vi "Values.vi"(11 "User in":refnum<class "User.lvclass">) -> (2 "Values":T1)   [LabVIEW 2022 SP3, in "Test.lvlib" / "User.lvclass"]
uses:
  User.lvclass
  Values.ctl
  User.lvclass/User.ctl
  <vilib>/IlluminatedG/IG Conditum/Conditum/Columns/String/String.lvclass/String.ctl
  <vilib>/IlluminatedG/IG Conditum/Conditum/Columns/Timestamp/Timestamp.lvclass/Timestamp.ctl
  <vilib>/IlluminatedG/IG Conditum/Conditum/Columns/Boolean/Boolean.lvclass/Boolean.ctl
  <vilib>/IlluminatedG/IG Conditum/Conditum/Columns/Integer/Integer.lvclass/Integer.ctl
  <vilib>/IlluminatedG/IG Conditum/Conditum/Columns/String/String.lvclass
  <vilib>/IlluminatedG/IG Conditum/Conditum/Columns/Timestamp/Timestamp.lvclass
  <vilib>/IlluminatedG/IG Conditum/Conditum/Columns/Boolean/Boolean.lvclass
  <vilib>/IlluminatedG/IG Conditum/Conditum/Columns/Integer/Integer.lvclass
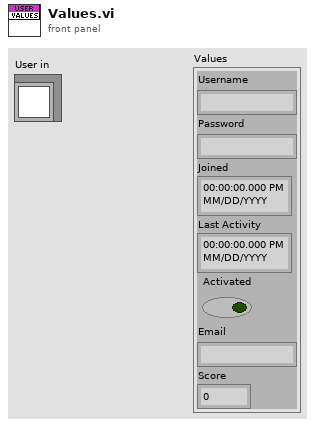
[diagram p1: front panel]
types:
  T1 = typedef "Test.lvlib/User.lvclass/Values.ctl" = cluster{"Username":string, "Password":string, "Joined":timestamp, "Last Activity":timestamp, "Activated":bool, "Email":string, "Score":i64}
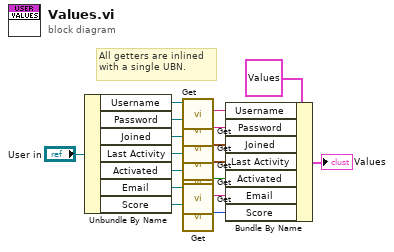
[diagram p0: block diagram]
diagram:
  # "All getters are inlined with a single UBN."
  n1 = Unbundle By Name("User in") -> ("Username"=w16:refnum<class "String.lvclass">, "Password"=w10:refnum<class "String.lvclass">, "Joined"=w15:refnum<class "Timestamp.lvclass">, "Last Activity"=w14:refnum<class "Timestamp.lvclass">, "Activated"=w13:refnum<class "Boolean.lvclass">, "Email"=w11:refnum<class "String.lvclass">, "Score"=w12:refnum<class "Integer.lvclass">)
  n2 = call <vilib>:"Get.vi"("String in"=w16) -> ("Value"=w8:string)  [unwired: 10 in]
  n3 = call <vilib>:"Get.vi"("String in"=w10) -> ("Value"=w7:string)  [unwired: 10 in]
  n4 = call <vilib>:"Get.vi"("Timestamp in"=w15) -> ("Value"=w6:timestamp)  [unwired: 10 in]
  n5 = call <vilib>:"Get.vi"("Timestamp in"=w14) -> ("Value"=w5:timestamp)  [unwired: 10 in]
  n6 = call <vilib>:"Get.vi"("Boolean in"=w13) -> ("Value"=w4:bool)  [unwired: 10 in]
  n7 = call <vilib>:"Get.vi"("String in"=w11) -> ("Value"=w3:string)  [unwired: 10 in]
  n8 = call <vilib>:"Get.vi"("Integer in"=w12) -> ("Value"=w2:i64)  [unwired: 10 in]
  n9 = Bundle By Name(cluster=T1 {"Username"="", "Password"="", "Joined"=timestamp(0 s since 1904-01-01), "Last Activity"=timestamp(0 s since 1904-01-01), "Activated"=FALSE, "Email"="", "Score"=0} ("Values"), "Username"=w8, "Password"=w7, "Joined"=w6, "Last Activity"=w5, "Activated"=w4, "Email"=w3, "Score"=w2) -> (→"Values":T1)
